vi "Digital UI Pins Logic.vi"(7 "Mode":enum16{"Initialize", "Process Changes"}(ring)=enum."Process Changes", 8 "error in":errorcluster, 9 "Initial Pin Names":string[](array[string]), 10 "OldVal":T1 {"Pin Value" format="%#_g V"}, 11 "NewVal":T1 {"Pin Value" format="%#_g V"}) -> (0 "error out":errorcluster, 3 "Updated Value":T1 {"Pin Value" format="%#_g V"})   [LabVIEW 2020]
uses:
  Controls/UI-Digital Pins.ctl
  Controls/UI-Digital Pin.ctl
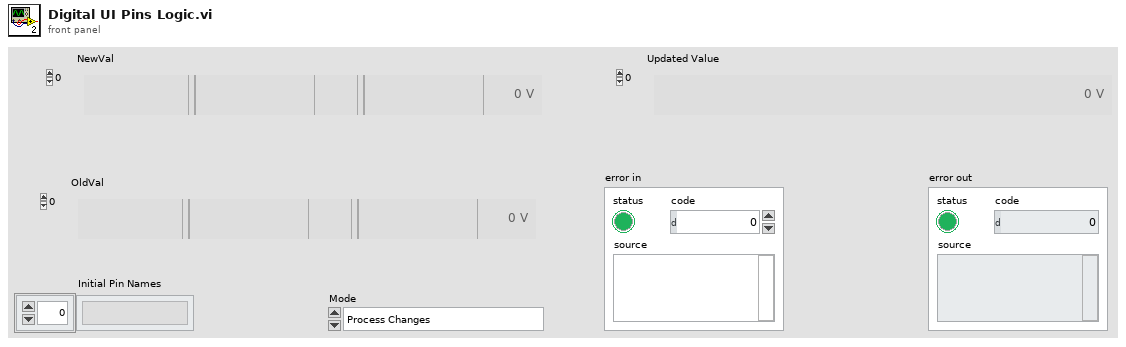
[diagram p1: front panel]
types:
  T1 = typedef "UI-Digital Pins.ctl" = T2[]
  T2 = typedef "UI-Digital Pin.ctl" = cluster{"IO Direction":u16, "Pin Direction":string, "DO Value":u16, "Pin Value":dbl, "Pin Index":string, "Pin Mode":string}
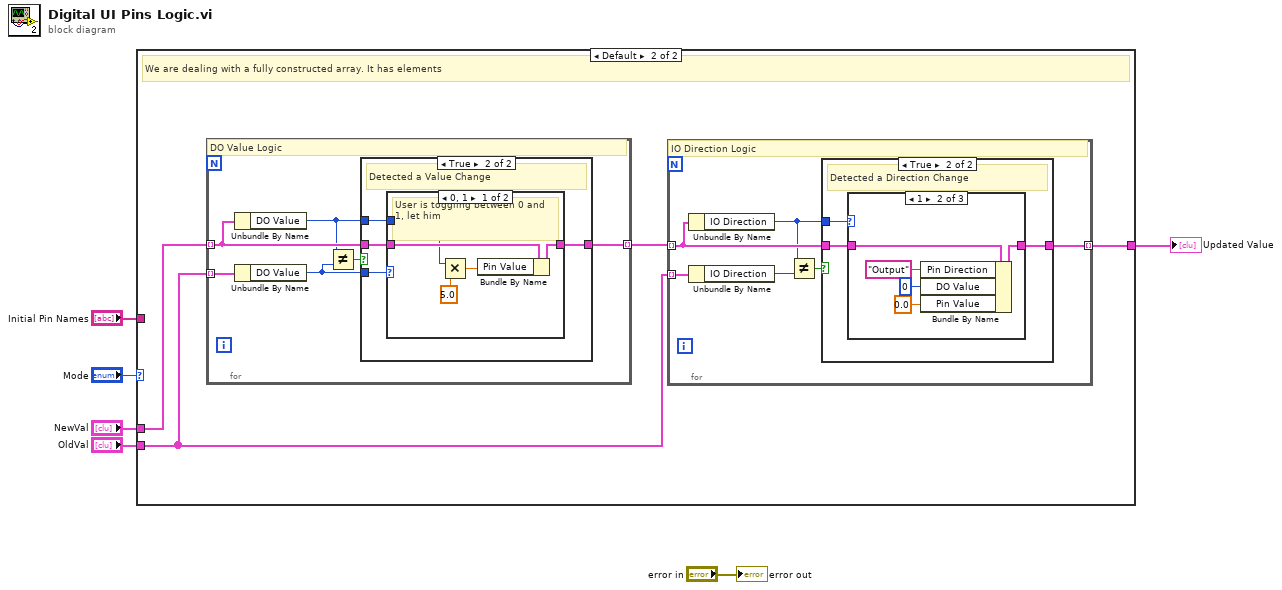
[diagram p0: block diagram]
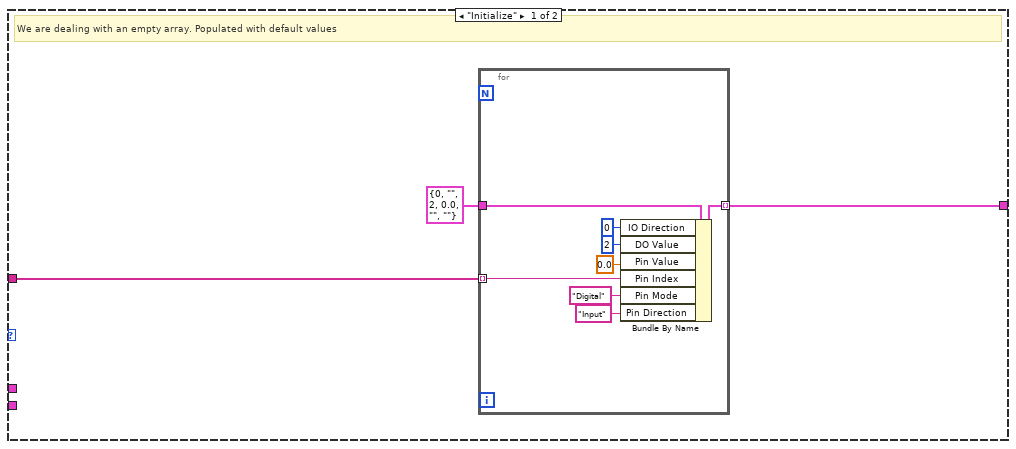
[diagram p2: hidden frame]
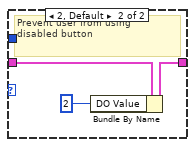
[diagram p4: hidden frame]
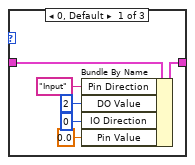
[diagram p6: hidden frame]
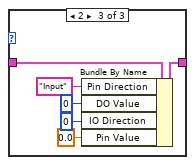
[diagram p7: hidden frame]
diagram:
  n1 = case shown="Default" "Mode" {
    tunnel: [w9 w21] -> w6
    tunnel: "OldVal" -> [_ w19]
    tunnel: "NewVal" -> [_ w18]
    tunnel: "Initial Pin Names" -> [w7 _]
    frame "Initialize" {
      # "We are dealing with an empty array. Populated with default values"
      n2 = for {
        tunnel: T2 {"IO Direction"=0, "Pin Direction"="", "DO Value"=2, "Pin Value"=0.0, "Pin Index"="", "Pin Mode"=""} ("Cluster") -> [w17]
        tunnel: [w16] -> w9 mode=indexing
        tunnel: w7 -> [w10] mode=indexing
        n3 = Bundle By Name(cluster=w17, "IO Direction"=u16 0, "DO Value"=u16 2, "Pin Value"=0.0 ("AI Value"), "Pin Index"=w10, "Pin Mode"="Digital", "Pin Direction"="Input") -> (w16:T2)
      }
    }
    frame Default {
      # "We are dealing with a fully constructed array. It has elements"
      n4 = for {
        tunnel: w18 -> [w26] mode=indexing
        tunnel: [w27] -> w20 mode=indexing
        tunnel: w19 -> [w25] mode=indexing
        # "DO Value Logic"
        n5 = Unbundle By Name(w26) -> ("DO Value"=w22:u16)
        n6 = Unbundle By Name(w25) -> ("DO Value"=w23:u16)
        n7 = Not Equal?(x=w22, y=w23) -> (x != y?=w24:bool)
        n8 = case shown="True" w24 {
          tunnel: [w28 w32] -> w27
          tunnel: w26 -> [w28 w31]
          tunnel: w23 -> [_ w30]
          tunnel: w22 -> [_ w29]
          frame False {
            # "Pin has same DO Value"
          }
          frame True {
            # "Detected a Value Change"
            n9 = case shown="0, 1" w30 {
              tunnel: [w36 w39] -> w32
              tunnel: w31 -> [w37 w40]
              tunnel: w29 -> [w33 _]
              frame 0, 1 {
                # "User is toggling between 0 and 1, let him"
                n10 = Multiply(x=w33, y=5.0) -> (x*y=w35:dbl)
                n11 = Bundle By Name(cluster=w37, "Pin Value"=w35) -> (w36:T2)
              }
              frame 2, Default {
                # "Prevent user from using\ndisabled button"
                n12 = Bundle By Name(cluster=w40, "DO Value"=u16 2) -> (w39:T2)
              }
            }
          }
        }
      }
      n13 = for {
        tunnel: w20 -> [w45] mode=indexing
        tunnel: [w46] -> w21 mode=indexing
        tunnel: w19 -> [w44] mode=indexing
        # "IO Direction Logic"
        n14 = Unbundle By Name(w45) -> ("IO Direction"=w42:u16)
        n15 = Unbundle By Name(w44) -> ("IO Direction"=w43:u16)
        n16 = Not Equal?(x=w42, y=w43) -> (x != y?=w41:bool)
        n17 = case shown="True" w41 {
          tunnel: w42 -> [_ w50]
          tunnel: [w47 w49] -> w46
          tunnel: w45 -> [w47 w48]
          frame False {
            # "Pin has same direction"
          }
          frame True {
            # "Detected a Direction Change"
            n18 = case shown="1" w50 {
              tunnel: [w55 w60 w66] -> w49
              tunnel: w48 -> [w56 w61 w67]
              frame 0, Default {
                n19 = Bundle By Name(cluster=w56, "Pin Direction"="Input", "DO Value"=u16 2, "IO Direction"=u16 0, "Pin Value"=0.0) -> (w55:T2)
              }
              frame 1 {
                n20 = Bundle By Name(cluster=w61, "Pin Direction"="Output", "DO Value"=u16 0, "Pin Value"=0.0) -> (w60:T2)
              }
              frame 2 {
                n21 = Bundle By Name(cluster=w67, "Pin Direction"="Input", "DO Value"=u16 0, "IO Direction"=u16 0, "Pin Value"=0.0) -> (w66:T2)
              }
            }
          }
        }
      }
    }
  }
  "Updated Value" <- w6
  "error out" <- "error in"
